vi "AB_Illegal_Function_Name_Error.vi"(11 "error string in":string) -> (3 "error string out":string)   [LabVIEW 2020]
uses:
  <resource>/Framework/Providers/Common/provcom_StringGlobals.vi
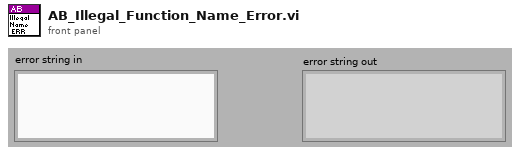
[diagram p1: front panel]
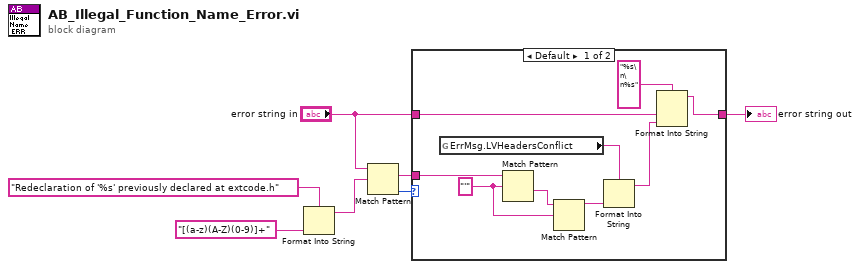
[diagram p0: block diagram]
diagram:
  n1 = Format Into String(format string="Redeclaration of '%s' previously declared at extcode.h" ("regular expression"), "[(a-z)(A-Z)(0-9)]+") -> (resulting string=w5:string)  [unwired: 2 in, 1 out]
  n2 = Match Pattern(string="error string in", regular expression=w5) -> (match substring=w3:string, offset past match=w4:i32)  [unwired: 1 in, 2 out]
  n3 = case shown="Default" w4 {
    tunnel: w3 -> [w16 _]
    tunnel: [w9 w17] -> w2
    tunnel: "error string in" -> [w11 w17]
    frame Default {
      w14 = "'" ("search string/char (-)")
      n4 = global read "provcom_StringGlobals.vi" "ErrMsg.LVHeadersConflict"() -> (w8:string)
      n5 = Match Pattern(string=w16, regular expression=w14) -> (after substring=w15:string)  [unwired: 1 in, 3 out]
      n6 = Match Pattern(string=w15, regular expression=w14) -> (before substring=w13:string)  [unwired: 1 in, 3 out]
      n7 = Format Into String(format string=w8, w13) -> (resulting string=w10:string)  [unwired: 2 in, 1 out]
      n8 = Format Into String(format string="%s\n\n%s", w11, w10) -> (resulting string=w9:string)  [unwired: 2 in, 1 out]
    }
    frame -1 {
    }
  }
  "error string out" <- w2
